vi "Open Spartan Database.vi"(8 "error in (no error)":errorcluster, 11 "DB Path (empty - use default)":path) -> (0 "error out":errorcluster, 3 "Connection Refnum":T1)   [LabVIEW 2011]
uses:
  Summitek EXT/ODBC/SQL Controls/Connection Refnum.ctl
  Summitek EXT/OpenG EXT/file/file.llb/Convert File Extension (Path)__ogtk.vi
  server lib/Spartan CONFIG Global.vi
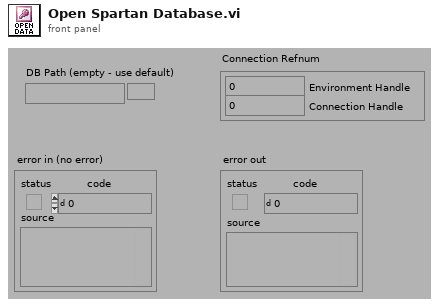
[diagram p1: front panel]
types:
  T1 = typedef "Connection Refnum.ctl" = cluster{"Environment Handle":i32, "Connection Handle":i32}
  T2 = typedef "Keyed Array.ctl" = cluster{"keys":string[], "values":string[]}
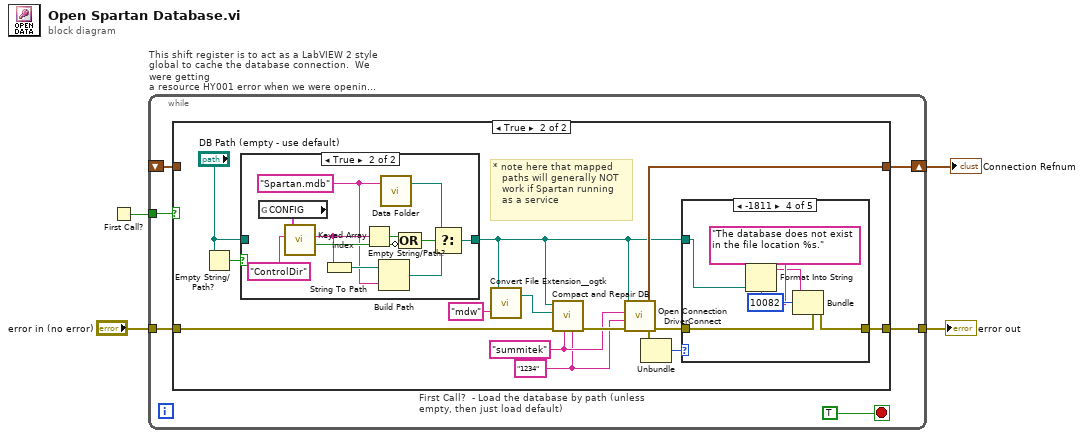
[diagram p0: block diagram]
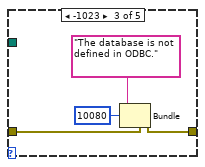
[diagram p6: hidden frame]
diagram:
  n1 = First Call?() -> (First Call?: T/F=w1:bool)
  n2 = while "This shift register is to act as a LabVIEW 2 style global to cache the database connection.  We were getting\na resource HY001 error when we were opening multiple handles to the database.  We now want to open\none handle when this VI is first called and then use this handle throughout Spartan instead of opening new handles all over." {
    tunnel: "error in (no error)" -> [w10]
    tunnel: [w9] -> w3
    shift-right: [w7] -> w2
    shift-left: _ -> [w8]
    tunnel: w1 -> [w5]
    stop <- TRUE stop-if-true
    n3 = case "First Call?  - Load the database by path (unless empty, then just load default)" shown="True" w5 {
      tunnel: w10 -> [w11 w17]
      tunnel: [w11 w21] -> w9
      tunnel: w8 -> [w12 _]
      tunnel: [w12 w20] -> w7
      frame False {
      }
      frame True {
        w14 = "1234" ("Username (\"\")")
        w15 = "summitek" ("Username (\"\")")
        # "* note here that mapped\n   paths will generally NOT\n   work if Spartan running\n   as a service"
        n4 = Empty String/Path?(string/path="DB Path (empty - use default)") -> (empty?=w23:bool)
        n5 = case shown="True" w23 {
          tunnel: "DB Path (empty - use default)" -> [w26 _]
          tunnel: [w26 w31] -> w13
          frame False {
          }
          frame True {
            w28 = "Spartan.mdb" ("name or relative path")
            n6 = global read "Spartan CONFIG Global.vi" "CONFIG"() -> (w37:T2)
            n7 = call "Keyed Array Index.vi"("key"="ControlDir", "array in"=w37) -> ("valid key"=w34:bool, "value"=w30:string)  [unwired: 2 in, 2 out]
            n8 = String To Path(string=w30) -> (path=w29:path)
            n9 = Empty String/Path?(string/path=w30) -> (empty?=w35:bool)
            n10 = Build Path(base path=w29, name or relative path=w28) -> (appended path=w27:path)
            n11 = call "Data Folder.vi"("Relative Path (\"\" - Folder)"=w28) -> ("Data Folder"=w32:path)  [unwired: 2 in]
            n12 = Compound Arithmetic op=OR(w35, invert w34) -> (w33:bool)
            n13 = Select(t=w32, s=w33, f=w27) -> (s? t:f=w31:path)
          }
        }
        n14 = call-poly "Convert File Extension__ogtk.vi"("new ending (none)"="mdw", "file name"=w13) -> ("new filename"=w19:path)  [unwired: 1 out]
        n15 = call "Compact and Repair DB.vi"("password (\"\")"=w14, "username (\"\")"=w15, "error in (no error)"=w17, "Workgroup DB (none)"=w19, "Database Path (empty)"=w13) -> ("error out"=w16:errorcluster)  [unwired: 6 out]
        n16 = call "Open Connection DriverConnect.vi"("error in (no error)"=w16, "Password (\"\")"=w14, "Username (\"\")"=w15, "ODBC Database (\"\")"=w13) -> ("error out"=w25:errorcluster, "Connection Refnum"=w20:T1)  [unwired: 3 out]
        n17 = Unbundle(w25) -> ("code"=w24:i32)  [unwired: 2 out]
        n18 = case shown="-1811" w24 {
          tunnel: [w38 w39 w43 w49 w50] -> w21
          tunnel: w25 -> [w38 w39 w42 w48 w50]
          tunnel: w13 -> [_ _ _ w45 _]
          frame 0 {
          }
          frame Default {
          }
          frame -1023 {
            n19 = Bundle(cluster=w42, "code"=10080, "source"="The database is not defined in ODBC.") -> (w43:errorcluster)  [unwired: 1 out]
          }
          frame -1811 {
            n20 = Format Into String(format string="The database does not exist in the file location %s." ("source"), w45) -> (resulting string=w44:string)  [unwired: 2 in, 1 out]
            n21 = Bundle(cluster=w48, "code"=10082, "source"=w44) -> (w49:errorcluster)  [unwired: 1 out]
          }
          frame 1 {
          }
        }
      }
    }
  }
  "Connection Refnum" <- w2
  "error out" <- w3
